vi "LPF2_Sensors.vi"() -> ()   [LabVIEW 2016]
uses:
  VIs/uPythonX/uPythonX.xctl
panel:
  in  "Talking BLE with a WeDo":T1(xcontrol)={"VISA Refnum in"="ASRL73::INSTR", "Python Code"="import hub, utime\n\ndef IDWeDo(devices):\n     reply = False\n     for device in devices:\n          service_id = device[\"service_id\"]\n          if service_id.find('00001623') >= 0:\n               print(service_id)\n               reply = True\n     return reply\n               \ndef dump_data(d):\n    print(\"CB z:\", ' '.join(['0x%02X ' % (byte) for byte in d]))\n\ndef connect_callback(a):\n     print('Connection complete: {0}'.format(a))\n          \nhub.ble.mac()\n\nhub.ble.rssi(-50)\nhub.ble.scan(10)\nf = hub.ble.scan_result()\n\nwhile not IDWeDo(f):\n     f = hub.ble.scan_result()\n     utime.sleep(0.2)\n\nhub.ble.callback(connect_callback)\n\ng = hub.ble.connect(0)\n\nutime.sleep(10)\n\npink = bytes([0x06, 0x04, 0x01, 0x01])  \n#06 is the port number (internal LED), 04 is the command number (change light color), 01 is the command size (only 1 argument), and 01 is the command value (color)\ng.send(pink)\n\ng.callback(dump_data)\n\ng.subscribe()\n\nutime.sleep(10)\n\ng.unsubscribe()\n\nf.disconnect()\n\n"}
  in  "ReadingWeDoSensor":T1(xcontrol)={"VISA Refnum in"="ASRL104::INSTR", "Python Code"="import machine,utime\n\nuart = machine.UART(1)\nrxPin = 'Y2'\n\ndef WaitForDip():\n     rx = machine.Pin(rxPin, machine.Pin.IN)\n     waiting = True\n     while waiting:\n          while not rx.value():\n               utime.sleep_ms(10)\n           starttime = utime.time()\n           while  rx.value():\n                utime.sleep_ms(10)\n            if (utime.time()-starttime > 400):\n                 waiting = False\n                 \ndef waitForCode():\n     while True:\n          length = uart.any()\n          if length > 0:\n                    print(uart.read(uart.any()))\n          utime.sleep(0.2)\n\n# machine.Pin(self.txPin, machine.Pin.OUT)\n#          self.rx = machine.Pin(self.rxPin, machine.Pin.IN)\n #         self.tx.value(0)\n#          utime.sleep_ms(500)\n#          self.tx.value(1)\n\nWaitForDip()\nuart.init(baudrate=2400, bits=8, parity=None, stop=1)\n          \nwaitForCode()\n\n# test\n"}
  # "3.3 V"
  # "GRND"
  # "Blue"
  # "Green"
  # "Yellow"
  # "Red"
  # "Orange"
  # "Magenta"
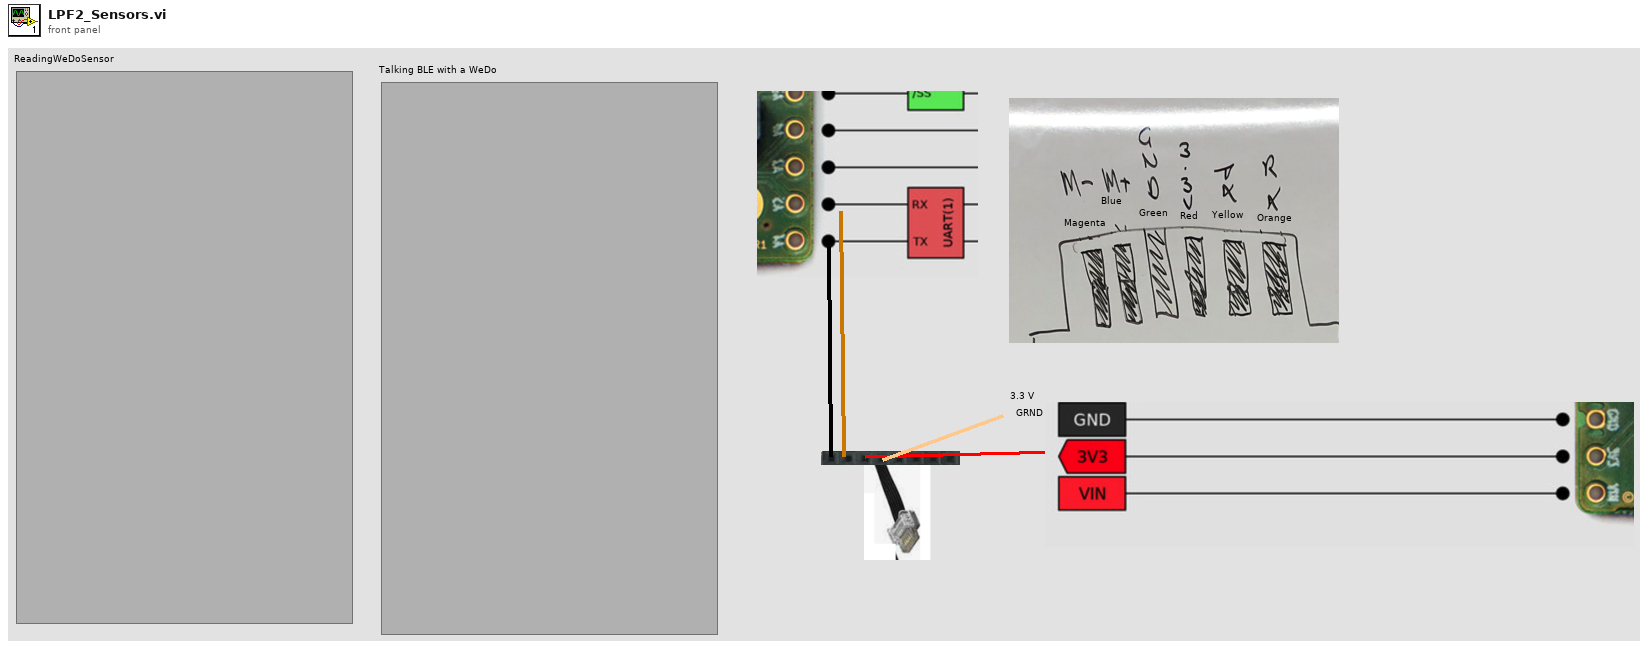
[diagram p1: front panel]
types:
  T1 = cluster{"VISA Refnum in":refnum<visa-resource-name>, "Python Code":string}
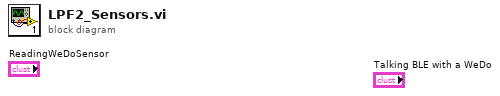
[diagram p0: block diagram]
diagram:
